vi "GuiUpdate.vi"(7 "GuiRef":T2={"StringOut"=refnum, "AbortOnFail"=refnum, "SN"=refnum, "SN_Length"=refnum, "TestResult"=refnum, "CycleTime"=refnum, "ErrorCode"=refnum, "UUTStatus"=refnum, "DataBaseEnable?"=refnum, "DUTModel"=refnum, "FixtureID"=refnum, "OperatorID"=refnum, "SNReady"=refnum, "StopSlot"=refnum, "NextStep"=refnum, "PassYeild"=refnum, "Failed"=refnum, "Passed"=refnum, "Tested"=refnum, "TestItemsCtl"={"StepName"="", "TestEnable"=FALSE, "LoopCount"=0, "StopOnFail"=FALSE, "Index"=0, "TestName"="", "通道"="", "参数"="", "TimeStart"=0}, "ProcessBar"=refnum, "Slot"=enum."Slot1", "Row"=3, "States"=refnum, "TestMode"=refnum, "循环次数-DUT"=refnum, "波形图"=refnum, "产品型号"=refnum, "子面板"=refnum, "测试失败项目"=refnum, "测试结果"=refnum, "DUT"=refnum, "Starttime"=refnum, "SlotReady"=refnum, "版本信息"=refnum, "WIFI_1"=refnum, "WIFI_2"=refnum, "直通率"=refnum, "卡1开卡结果"=refnum, "卡2开卡结果"=refnum}, 8 "error in":errorcluster, 9 "States":T1=enum."PostUUT") -> (0 "error out":errorcluster, 2 "PASS/FAIL":bool)   [LabVIEW 2013]
uses:
  SysControl/Reference.ctl
  SysControl/TestItemsCTL.ctl
  SysControl/Slot.ctl
  SysControl/States.ctl
  SysControl/LEDState.ctl
  SysControl/Setup.ctl
  SourceCode/GlobalValue.vi
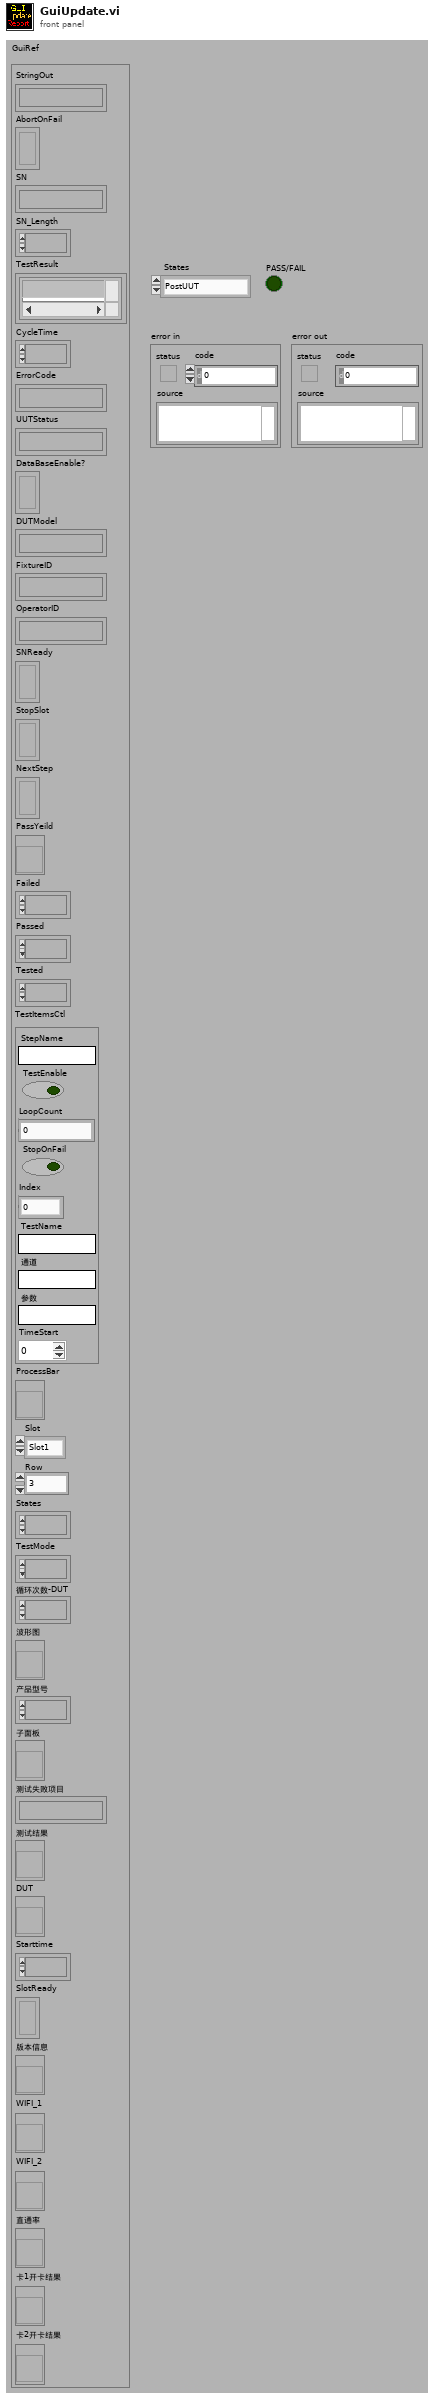
[diagram p1: front panel]
types:
  T1 = typedef "States.ctl" = enum16{"Init", "PreUUT", "Idle", "SetUp", "TestSequence", "PostUUT", "StopTest", "Debug Mode", "Selection Mode", "Loop Mode", "Error", "Wait"}
  T2 = typedef "Reference.ctl" = cluster{"StringOut":refnum<vi>, "AbortOnFail":refnum<vi>, "SN":refnum<vi>, "SN_Length":refnum<vi>, "TestResult":refnum<vi>, "CycleTime":refnum<vi>, "ErrorCode":refnum<vi>, "UUTStatus":refnum<vi>, "DataBaseEnable?":refnum<vi>, "DUTModel":refnum<vi>, "FixtureID":refnum<vi>, "OperatorID":refnum<vi>, "SNReady":refnum<vi>, "StopSlot":refnum<vi>, "NextStep":refnum<vi>, "PassYeild":refnum<vi>, "Failed":refnum<vi>, "Passed":refnum<vi>, "Tested":refnum<vi>, "TestItemsCtl":T3, "ProcessBar":refnum<vi>, "Slot":T4, "Row":u32, "States":refnum<vi>, "TestMode":refnum<vi>, "循环次数-DUT":refnum<vi>, "波形图":refnum<vi>, "产品型号":refnum<vi>, "子面板":refnum<vi>, "测试失败项目":refnum<vi>, "测试结果":refnum<vi>, "DUT":refnum<vi>, "Starttime":refnum<vi>, "SlotReady":refnum<vi>, "版本信息":refnum<vi>, "WIFI_1":refnum<vi>, "WIFI_2":refnum<vi>, "直通率":refnum<vi>, "卡1开卡结果":refnum<vi>, "卡2开卡结果":refnum<vi>}
  T3 = typedef "TestItemsCTL.ctl" = cluster{"StepName":string, "TestEnable":bool, "LoopCount":i32, "StopOnFail":bool, "Index":u32, "TestName":string, "通道":string, "参数":string, "TimeStart":u32}
  T4 = typedef "Slot.ctl" = enum16{"Slot1", "Slot2", "Slot3", "Slot4"}
  T5 = enum8{"Enabled", "Disabled", "Disabled and Grayed Out"}
  T6 = typedef "LEDState.ctl" = enum16{"默认", "闪烁", "停止闪烁", "真", "假"}
  T7 = typedef "Setup.ctl" = cluster{"TestedNum":u32, "PassedNum":u32, "FailedNum":u32, "Slot1TestedNum":u32, "Slot2TestedNum":u32, "Slot3TestedNum":u32, "Slot4TestedNum":u32, "GuiVer":string, "LimitFileVer":string, "Login Name":string, "Password":string, "SN_Head":string, "SN_Length":i32, "AbortOnFail":bool, "DataBaseEnable?":bool, "FixtureID":string, "ShowSkipStep?":bool}
  T8 = typedef "TestMode.ctl" = enum16{"Production Mode", "Selection Mode", "Debug Mode", "Loop Mode", "Stop Test"}
  T9 = enum16{"Production Mode", "Selection Mode", "Debug Mode", "Loop Mode", "Stop Test"}
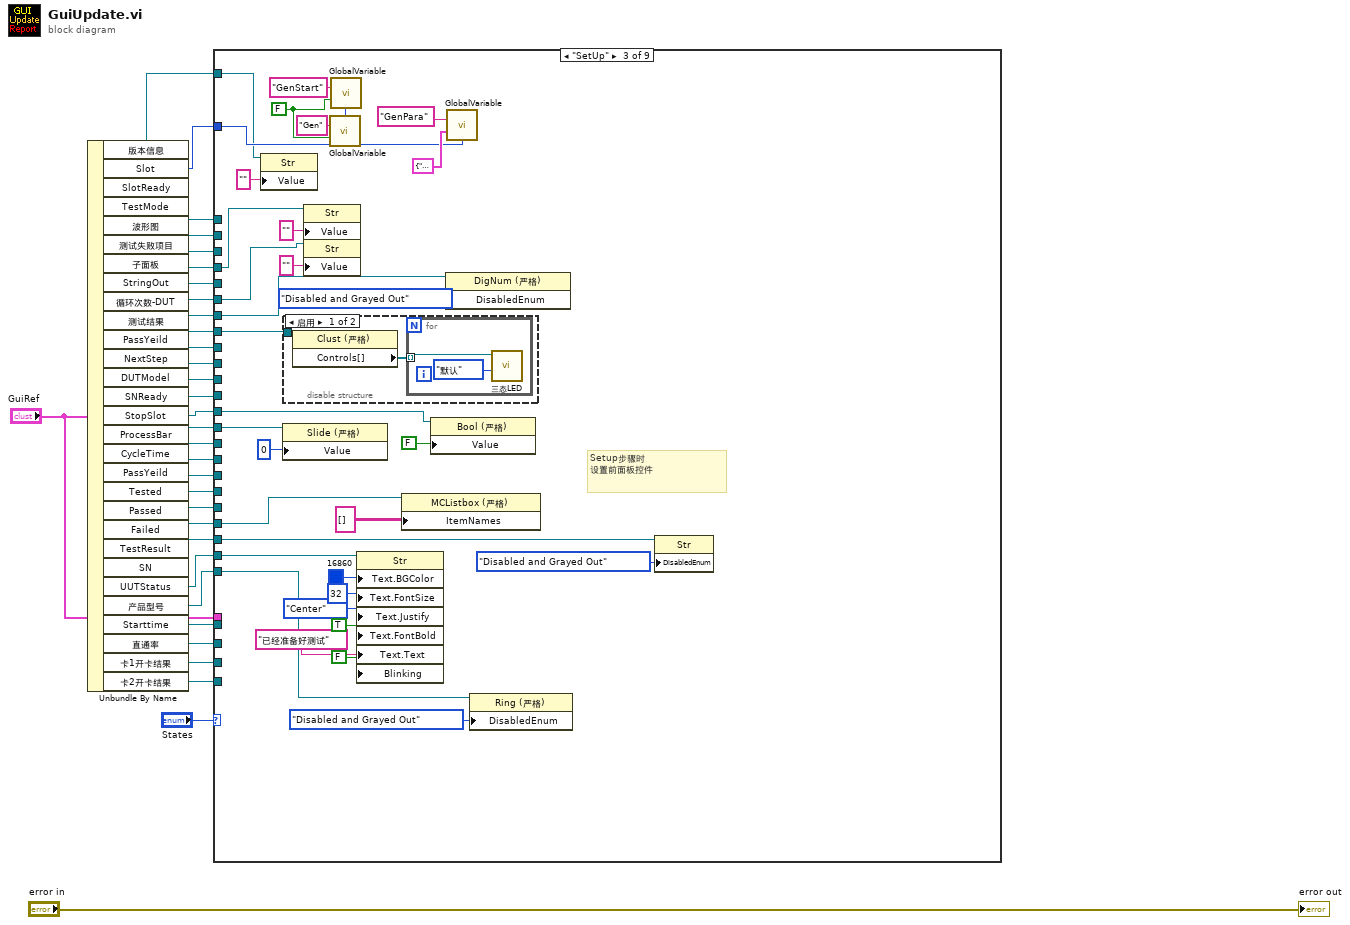
[diagram p0: block diagram]
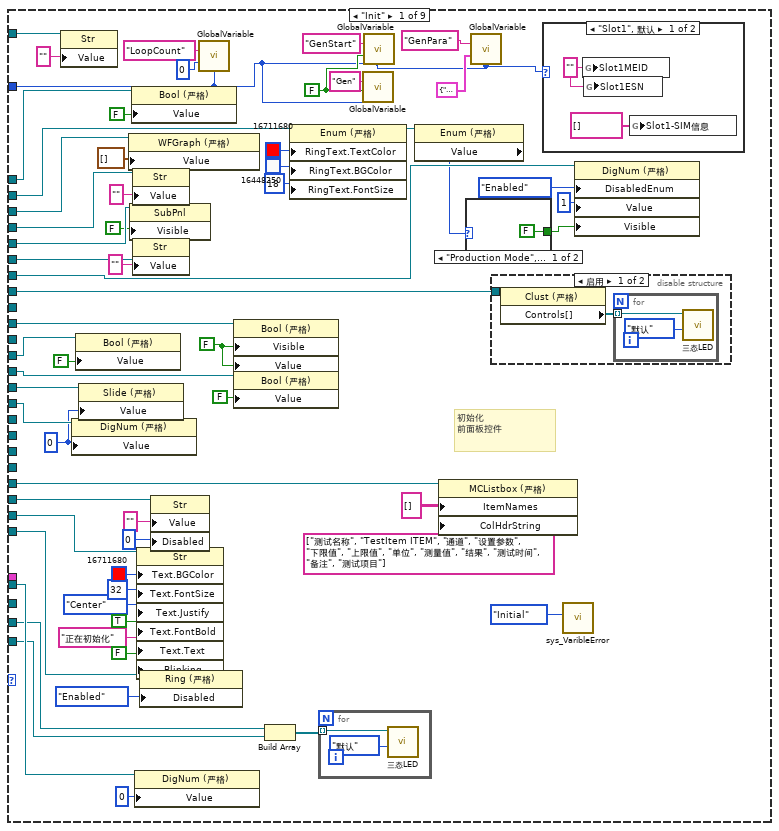
[diagram p2: hidden frame]
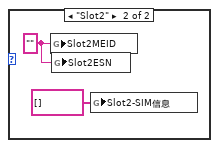
[diagram p3: hidden frame]
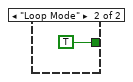
[diagram p4: hidden frame]
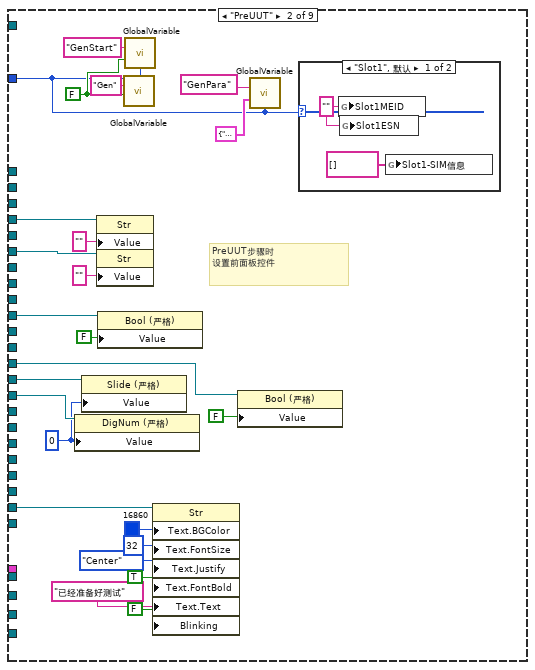
[diagram p6: hidden frame]
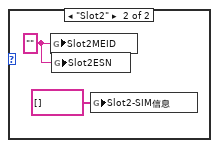
[diagram p7: hidden frame]
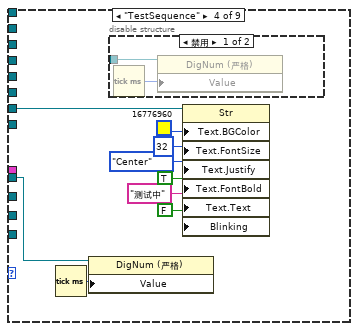
[diagram p9: hidden frame]
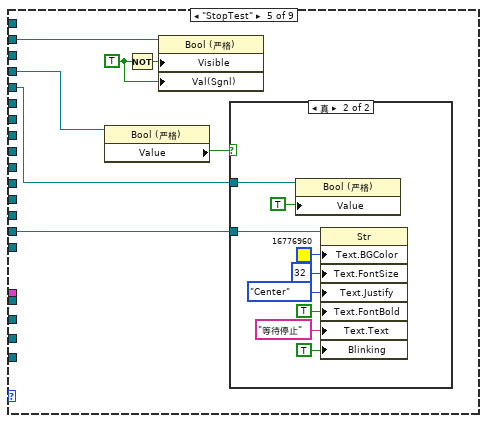
[diagram p11: hidden frame]
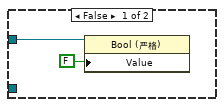
[diagram p12: hidden frame]
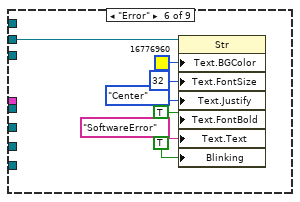
[diagram p13: hidden frame]
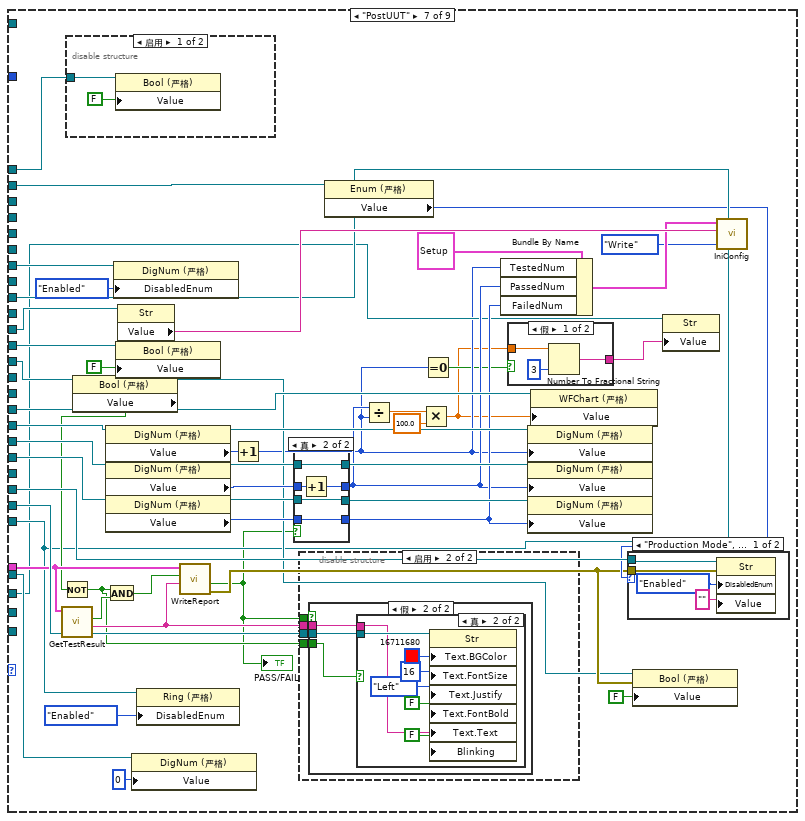
[diagram p14: hidden frame]
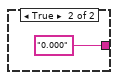
[diagram p15: hidden frame]
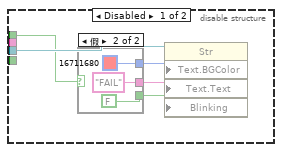
[diagram p18: hidden frame]
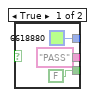
[diagram p19: hidden frame]
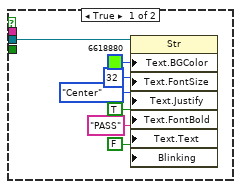
[diagram p20: hidden frame]
diagram:
  n1 = Unbundle By Name("GuiRef") -> ("版本信息"=w4:refnum<vi>, "Slot"=w5:T4, "SlotReady"=w6:refnum<vi>, "TestMode"=w8:refnum<vi>, "波形图"=w9:refnum<vi>, "测试失败项目"=w10:refnum<vi>, "子面板"=w11:refnum<vi>, "StringOut"=w12:refnum<vi>, "循环次数-DUT"=w15:refnum<vi>, "测试结果"=w16:refnum<vi>, "PassYeild"=w18:refnum<vi>, "NextStep"=w19:refnum<vi>, "DUTModel"=w21:refnum<vi>, "SNReady"=w24:refnum<vi>, "StopSlot"=w14:refnum<vi>, "ProcessBar"=w23:refnum<vi>, "CycleTime"=w22:refnum<vi>, "PassYeild"=w28:refnum<vi>, "Tested"=w27:refnum<vi>, "Passed"=w26:refnum<vi>, "Failed"=w25:refnum<vi>, "TestResult"=w30:refnum<vi>, "SN"=w32:refnum<vi>, "UUTStatus"=w31:refnum<vi>, "产品型号"=w13:refnum<vi>, "Starttime"=w7:refnum<vi>, "直通率"=w3:refnum<vi>, "卡1开卡结果"=w2:refnum<vi>, "卡2开卡结果"=w1:refnum<vi>)
  n2 = case shown="\"SetUp\"" "States" {
    tunnel: w32 -> [w91 _ w160 _ _ _ w231 _ _]
    tunnel: w31 -> [w64 w117 w146 w172 w187 w199 w256 _ w340]
    tunnel: w30 -> [w84 _ w163 _ _ _ _ _ _]
    tunnel: w28 -> [_ _ _ _ _ _ w242 _ w321]
    tunnel: w27 -> [_ _ _ _ _ _ w254 _ w337]
    tunnel: w26 -> [_ _ _ _ _ _ w253 _ w336]
    tunnel: w25 -> [_ _ _ _ _ _ w255 _ w338]
    tunnel: w23 -> [w90 w128 w165 _ _ _ _ _ _]
    tunnel: w22 -> [w89 w127 _ _ _ _ _ _ _]
    tunnel: w24 -> [w87 _ _ _ w182 _ w241 _ w319]
    tunnel: w21 -> [_ _ _ _ _ _ w240 _ _]
    tunnel: "GuiRef" -> [_ _ _ _ _ _ w233 _ w318]
    tunnel: w19 -> [w86 w114 _ _ w185 _ _ _ _]
    tunnel: w18 -> [_ _ _ _ _ _ w232 _ _]
    tunnel: w16 -> [w73 _ w158 _ _ _ _ _ _]
    tunnel: w15 -> [w81 _ w162 _ _ _ w230 _ _]
    tunnel: w14 -> [w80 w112 w142 _ w183 _ w228 _ _]
    tunnel: w13 -> [w78 _ w157 _ _ _ w212 _ _]
    tunnel: w12 -> [w76 w124 w155 _ _ _ _ _ _]
    tunnel: w11 -> [w75 _ _ _ _ _ _ _ _]
    tunnel: w10 -> [w71 w122 w153 _ _ _ _ _ _]
    tunnel: w9 -> [w62 _ _ _ _ _ _ _ _]
    tunnel: w8 -> [w57 _ _ _ _ _ w221 _ _]
    tunnel: w7 -> [w54 _ _ w170 _ _ w226 _ _]
    tunnel: w6 -> [w49 _ _ _ _ _ w222 _ w316]
    tunnel: w5 -> [w38 w106 w136 _ _ _ _ _ _]
    tunnel: w4 -> [w37 _ w134 _ _ _ _ _ _]
    tunnel: w3 -> [_ _ _ _ _ _ w210 _ _]
    tunnel: w2 -> [w34 _ _ _ _ _ _ _ _]
    tunnel: w1 -> [w33 _ _ _ _ _ _ _ _]
    frame "Init" {
      w44 = FALSE ("Value")
      w56 = FALSE ("可见")
      w88 = 0 ("Value")
      # "初始化\n前面板控件"
      n3 = property class="Str"(reference=w37, "Value"="" ("值")) -> ()  [unwired: 1 in, 2 out]
      n4 = property class="DigNum (严格)"(reference=w89, "Value"=w88) -> ()  [unwired: 1 in, 2 out]
      n5 = property class="Bool (严格)"(reference=w87, "Value"=FALSE) -> ()  [unwired: 1 in, 2 out]
      n6 = property class="Slide (严格)"(reference=w90, "Value"=w88) -> ()  [unwired: 1 in, 2 out]
      n7 = property class="WFGraph (严格)"(reference=w62, "Value"=waveform(dbl)[] [] ("Fail项波形图2")) -> ()  [unwired: 1 in, 2 out]
      n8 = property class="SubPnl"(reference=w75, "Visible"=FALSE ("可见")) -> ()  [unwired: 1 in, 2 out]
      n9 = property class="Bool (严格)"(reference=w49, "Value"=FALSE) -> ()  [unwired: 1 in, 2 out]
      n10 = property class="Str"(reference=w71, "Value"="" ("值")) -> ()  [unwired: 1 in, 2 out]
      n11 = property class="Str"(reference=w76, "Value"="" ("值")) -> ()  [unwired: 1 in, 2 out]
      n12 = property class="DigNum (严格)"(reference=w54, "Value"=u32 0 ("值")) -> ()  [unwired: 1 in, 2 out]
      n13 = property on="Property Node" class="Str"(reference=w64, "Text.BGColor"=u32 16711680 ("Color Box 2"), "Text.FontSize"=u32 32 ("文本.字体:字号"), "Text.Justify"=enum16{"Left", "Center", "Right"}."Center" ("文本.调整"), "Text.FontBold"=TRUE ("文本.字体:粗体"), "Text.Text"="正在初始化", "Blinking"=FALSE) -> ()  [unwired: 1 in, 2 out]
      n14 = property class="Ring (严格)"(reference=w78, "Disabled"=T5."Enabled" ("禁用")) -> ()  [unwired: 1 in, 2 out]
      n15 = property class="Str"(reference=w91, "Value"="", "Disabled"=u8 0) -> ()  [unwired: 1 in, 2 out]
      n16 = call "GlobalVariable.vi"("Name"="LoopCount", "ValueIn"=0 ("值"), "Slot"=w38) -> ()  [unwired: 9 in, 4 out]
      n17 = property class="Bool (严格)"(reference=w86, "Visible"=w56, "Value"=w56) -> ()  [unwired: 1 in, 2 out]
      n18 = property class="Bool (严格)"(reference=w80, "Value"=FALSE) -> ()  [unwired: 1 in, 2 out]
      n19 = Build Array(w34, w33) -> (w35:refnum<vi>[])
      n20 = property on="属性节点" class="Enum (严格)"(reference=w57, "RingText.TextColor"=u32 16711680 ("Color Box"), "RingText.BGColor"=u32 16448250 ("Color Box"), "RingText.FontSize"=u32 18 ("下拉列表文本.字体:字号")) -> (reference out=w43:refnum<vi>)  [unwired: 1 in, 1 out]
      n21 = for "For循环" {
        tunnel: w35 -> [w94] mode=indexing
        n22 = call "三态LED.vi"("State"=LEDState."默认", "Ctl引用句柄"=w94) -> ()  [unwired: 4 in, 2 out]
      }
      n23 = call "GlobalVariable.vi"("Name"="Gen", "ValueIn"=w44, "Slot"=w38) -> ()  [unwired: 9 in, 4 out]
      n24 = call "GlobalVariable.vi"("Name"="GenStart", "ValueIn"=w44, "Slot"=w38) -> ()  [unwired: 9 in, 4 out]
      n25 = property on="属性节点" class="Enum (严格)"(reference=w43) -> ("Value"=w42:T8)  [unwired: 1 in, 2 out]
      n26 = property class="MCListbox (严格)"(reference=w84, "ItemNames"=string[][] [] ("项名"), "ColHdrString"=string[] ["测试名称", "TestItem ITEM", "通道", "设置参数", "下限值", "上限值", "单位", "测量值", "结果", "测试时间", "备注", "测试项目"] ("列首字符串[]")) -> ()  [unwired: 1 in, 2 out]
      n27 = case shown="\"Production Mode\", 默认" w42 {
        tunnel: [FALSE ("可见") TRUE ("可见")] -> w41
        frame "Production Mode", Default {
        }
        frame "Loop Mode" {
        }
      }
      n28 = call "GlobalVariable.vi"("Name"="GenPara", "ValueIn"=cluster{"CH":tag, "Freq":dbl, "AMP":dbl} {"CH"="Dev1/ao1", "Freq"=0.0, "AMP"=0.0} ("Paras 2"), "Slot"=w38) -> ()  [unwired: 9 in, 4 out]
      n29 = disable-structure shown="启用" {
        disable-tunnel: w73 -> [w103 _]
        frame Enabled {
          n30 = property class="Clust (严格)"(reference=w103) -> ("Controls[]"=w102:refnum<vi>[])  [unwired: 1 in, 2 out]
          n31 = for "For循环" {
            tunnel: w102 -> [w104] mode=indexing
            n32 = call "三态LED.vi"("State"=LEDState."默认", "Ctl引用句柄"=w104) -> ()  [unwired: 4 in, 2 out]
          }
        }
        frame Disabled {
        }
      }
      n33 = case shown="\"Slot1\", 默认" w38 {
        frame "Slot1", Default {
          w97 = "" ("Slot2MEID")
          n34 = global write "GlobalValue.vi" "Slot1MEID"(w97) -> ()
          n35 = global write "GlobalValue.vi" "Slot1ESN"(w97) -> ()
          n36 = global write "GlobalValue.vi" "Slot1-SIM信息"(string[] [] ("Slot2-SIM信息")) -> ()
        }
        frame "Slot2" {
          w99 = "" ("Slot2MEID")
          n37 = global write "GlobalValue.vi" "Slot2MEID"(w99) -> ()
          n38 = global write "GlobalValue.vi" "Slot2ESN"(w99) -> ()
          n39 = global write "GlobalValue.vi" "Slot2-SIM信息"(string[] [] ("Slot2-SIM信息")) -> ()
        }
      }
      n40 = call "sys_VaribleError.vi"("Operation"=enum16{"Initial", "Collect"}."Initial") -> ()  [unwired: 10 in, 1 out]
      n41 = property class="DigNum (严格)"(reference=w81, "DisabledEnum"=T5."Enabled" ("禁用"), "Value"=1 ("值"), "Visible"=w41) -> ()  [unwired: 1 in, 2 out]
    }
    frame "PreUUT" {
      w109 = FALSE ("Value")
      w126 = 0 ("Value")
      # "PreUUT步骤时\n设置前面板控件"
      n42 = property class="DigNum (严格)"(reference=w127, "Value"=w126) -> ()  [unwired: 1 in, 2 out]
      n43 = property class="Slide (严格)"(reference=w128, "Value"=w126) -> ()  [unwired: 1 in, 2 out]
      n44 = property class="Str"(reference=w122, "Value"="" ("值")) -> ()  [unwired: 1 in, 2 out]
      n45 = property class="Str"(reference=w124, "Value"="" ("值")) -> ()  [unwired: 1 in, 2 out]
      n46 = property class="Bool (严格)"(reference=w114, "Value"=FALSE) -> ()  [unwired: 1 in, 2 out]
      n47 = call "GlobalVariable.vi"("Name"="Gen", "ValueIn"=w109) -> ()  [unwired: 10 in, 4 out]
      n48 = call "GlobalVariable.vi"("Name"="GenStart", "ValueIn"=w109, "Slot"=w106) -> ()  [unwired: 9 in, 4 out]
      n49 = property on="Property Node" class="Str"(reference=w117, "Text.BGColor"=u32 16860 ("Color Box 2"), "Text.FontSize"=u32 32 ("文本.字体:字号"), "Text.Justify"=enum16{"Left", "Center", "Right"}."Center" ("文本.调整"), "Text.FontBold"=TRUE ("文本.字体:粗体"), "Text.Text"="已经准备好测试", "Blinking"=FALSE) -> ()  [unwired: 1 in, 2 out]
      n50 = property class="Bool (严格)"(reference=w112, "Value"=FALSE) -> ()  [unwired: 1 in, 2 out]
      n51 = call "GlobalVariable.vi"("Name"="GenPara", "ValueIn"=cluster{"CH":tag, "Freq":dbl, "AMP":dbl} {"CH"="Dev1/ao1", "Freq"=0.0, "AMP"=0.0} ("Paras 2"), "Slot"=w106) -> ()  [unwired: 9 in, 4 out]
      n52 = case shown="\"Slot1\", 默认" w106 {
        frame "Slot1", Default {
          w131 = "" ("Slot2MEID")
          n53 = global write "GlobalValue.vi" "Slot1MEID"(w131) -> ()
          n54 = global write "GlobalValue.vi" "Slot1ESN"(w131) -> ()
          n55 = global write "GlobalValue.vi" "Slot1-SIM信息"(string[] [] ("Slot2-SIM信息")) -> ()
        }
        frame "Slot2" {
          w133 = "" ("Slot2MEID")
          n56 = global write "GlobalValue.vi" "Slot2MEID"(w133) -> ()
          n57 = global write "GlobalValue.vi" "Slot2ESN"(w133) -> ()
          n58 = global write "GlobalValue.vi" "Slot2-SIM信息"(string[] [] ("Slot2-SIM信息")) -> ()
        }
      }
    }
    frame "SetUp" {
      w139 = FALSE ("Value")
      # "Setup步骤时\n设置前面板控件"
      n59 = property class="Str"(reference=w134, "Value"="" ("值")) -> ()  [unwired: 1 in, 2 out]
      n60 = property class="Slide (严格)"(reference=w165, "Value"=0) -> ()  [unwired: 1 in, 2 out]
      n61 = disable-structure shown="启用" {
        disable-tunnel: w158 -> [w167 _]
        frame Enabled {
          n62 = property class="Clust (严格)"(reference=w167) -> ("Controls[]"=w166:refnum<vi>[])  [unwired: 1 in, 2 out]
          n63 = for "For循环" {
            tunnel: w166 -> [w168] mode=indexing
            n64 = call "三态LED.vi"("State"=LEDState."默认", "Ctl引用句柄"=w168) -> ()  [unwired: 4 in, 2 out]
          }
        }
        frame Disabled {
        }
      }
      n65 = property class="Str"(reference=w153, "Value"="" ("值")) -> ()  [unwired: 1 in, 2 out]
      n66 = property class="Str"(reference=w155, "Value"="" ("值")) -> ()  [unwired: 1 in, 2 out]
      n67 = call "GlobalVariable.vi"("Name"="Gen", "ValueIn"=w139, "Slot"=w136) -> ()  [unwired: 9 in, 4 out]
      n68 = call "GlobalVariable.vi"("Name"="GenStart", "ValueIn"=w139, "Slot"=w136) -> ()  [unwired: 9 in, 4 out]
      n69 = property on="Property Node" class="Str"(reference=w146, "Text.BGColor"=u32 16860 ("Color Box 2"), "Text.FontSize"=u32 32 ("文本.字体:字号"), "Text.Justify"=enum16{"Left", "Center", "Right"}."Center" ("文本.调整"), "Text.FontBold"=TRUE ("文本.字体:粗体"), "Text.Text"="已经准备好测试", "Blinking"=FALSE) -> ()  [unwired: 1 in, 2 out]
      n70 = property class="MCListbox (严格)"(reference=w163, "ItemNames"=string[][] [] ("项名")) -> ()  [unwired: 1 in, 2 out]
      n71 = property class="Bool (严格)"(reference=w142, "Value"=FALSE) -> ()  [unwired: 1 in, 2 out]
      n72 = property class="DigNum (严格)"(reference=w162, "DisabledEnum"=T5."Disabled and Grayed Out" ("禁用")) -> ()  [unwired: 1 in, 2 out]
      n73 = call "GlobalVariable.vi"("Name"="GenPara", "ValueIn"=cluster{"CH":tag, "Freq":dbl, "AMP":dbl} {"CH"="Dev1/ao1", "Freq"=0.0, "AMP"=0.0} ("Paras 2"), "Slot"=w136) -> ()  [unwired: 9 in, 4 out]
      n74 = property class="Ring (严格)"(reference=w157, "DisabledEnum"=T5."Disabled and Grayed Out" ("禁用")) -> ()  [unwired: 1 in, 2 out]
      n75 = property class="Str"(reference=w160, "DisabledEnum"=T5."Disabled and Grayed Out" ("禁用")) -> ()  [unwired: 1 in, 2 out]
    }
    frame "TestSequence" {
      n76 = Tick Count (ms)() -> (millisecond timer value=w171:u32)
      n77 = property class="DigNum (严格)"(reference=w170, "Value"=w171) -> ()  [unwired: 1 in, 2 out]
      n78 = disable-structure shown="禁用" {
        disable-tunnel: _ -> [w180 _]
        frame Disabled {
          n79 = Tick Count (ms)() -> (millisecond timer value=w179:u32)
          n80 = property on="Property Node" class="DigNum (严格)"(reference=w180, "Value"=w179) -> ()  [unwired: 1 in, 2 out]
        }
        frame Enabled {
        }
      }
      n81 = property on="Property Node" class="Str"(reference=w172, "Text.BGColor"=u32 16776960 ("Color Box 2"), "Text.FontSize"=u32 32 ("文本.字体:字号"), "Text.Justify"=enum16{"Left", "Center", "Right"}."Center" ("文本.调整"), "Text.FontBold"=TRUE ("文本.字体:粗体"), "Text.Text"="测试中", "Blinking"=FALSE) -> ()  [unwired: 1 in, 2 out]
    }
    frame "StopTest" {
      w184 = TRUE
      n82 = property class="Bool (严格)"(reference=w182) -> ("Value"=w181:bool)  [unwired: 1 in, 2 out]
      n83 = Not(x=w184) -> (.not. x?=w186:bool)
      n84 = property on="属性节点" class="Bool (严格)"(reference=w185, "Visible"=w186, "Val(Sgnl)"=w184) -> ()  [unwired: 1 in, 2 out]
      n85 = case shown="真" w181 {
        tunnel: w187 -> [_ w192]
        tunnel: w183 -> [w189 w191]
        frame False {
          n86 = property class="Bool (严格)"(reference=w189, "Value"=FALSE ("值")) -> ()  [unwired: 1 in, 2 out]
        }
        frame True {
          n87 = property class="Bool (严格)"(reference=w191, "Value"=TRUE ("值")) -> ()  [unwired: 1 in, 2 out]
          n88 = property on="Property Node" class="Str"(reference=w192, "Text.BGColor"=u32 16776960 ("Color Box 2"), "Text.FontSize"=u32 32 ("文本.字体:字号"), "Text.Justify"=enum16{"Left", "Center", "Right"}."Center" ("文本.调整"), "Text.FontBold"=TRUE ("文本.字体:粗体"), "Text.Text"="等待停止", "Blinking"=TRUE) -> ()  [unwired: 1 in, 2 out]
        }
      }
    }
    frame "Error" {
      n89 = property on="Property Node" class="Str"(reference=w199, "Text.BGColor"=u32 16776960 ("Color Box 2"), "Text.FontSize"=u32 32 ("文本.字体:字号"), "Text.Justify"=enum16{"Left", "Center", "Right"}."Center" ("文本.调整"), "Text.FontBold"=TRUE ("文本.字体:粗体"), "Text.Text"="SoftwareError", "Blinking"=TRUE) -> ()  [unwired: 1 in, 2 out]
    }
    frame "PostUUT" {
      n90 = call "GetTestResult.vi"("GuiRef"=w233) -> ("FailStep"=w227:string, "PASS/FAIL"=w218:bool)  [unwired: 3 in, 6 out]
      n91 = disable-structure shown="启用" {
        disable-tunnel: w222 -> [w265 _]
        frame Enabled {
          n92 = property class="Bool (严格)"(reference=w265, "Value"=FALSE ("值")) -> ()  [unwired: 1 in, 2 out]
        }
        frame Disabled {
        }
      }
      n93 = property class="Bool (严格)"(reference=w228) -> (reference out=w214:refnum<vi>, "Value"=w219:bool)  [unwired: 1 in, 1 out]
      n94 = Not(x=w219) -> (.not. x?=w216:bool)
      n95 = property on="Property Node" class="DigNum (严格)"(reference=w254) -> (reference out=w251:refnum<vi>, "Value"=w252:u32)  [unwired: 1 in, 1 out]
      n96 = property on="Property Node" class="DigNum (严格)"(reference=w253) -> (reference out=w247:refnum<vi>, "Value"=w250:u32)  [unwired: 1 in, 1 out]
      n97 = property on="Property Node" class="DigNum (严格)"(reference=w255) -> (reference out=w246:refnum<vi>, "Value"=w249:u32)  [unwired: 1 in, 1 out]
      n98 = And(x=w216, y=w218) -> (x .and. y?=w217:bool)
      n99 = property class="DigNum (严格)"(reference=w230, "DisabledEnum"=T5."Enabled" ("禁用")) -> ()  [unwired: 1 in, 2 out]
      n100 = property class="Bool (严格)"(reference=w241, "Value"=FALSE ("值")) -> ()  [unwired: 1 in, 2 out]
      n101 = property class="Str"(reference=w240) -> ("Value"=w239:string)  [unwired: 1 in, 2 out]
      n102 = property class="DigNum (严格)"(reference=w226, "Value"=u32 0 ("值")) -> ()  [unwired: 1 in, 2 out]
      n103 = property class="Ring (严格)"(reference=w212, "DisabledEnum"=T5."Enabled" ("禁用")) -> ()  [unwired: 1 in, 2 out]
      n104 = call "WriteReport.vi"("StepName"=w227, "Pass/Fail"=w217, "GuiRef"=w233) -> ("error out"=w215:errorcluster, "DBresult"=w211:bool)  [unwired: 6 in, 1 out]
      "PASS/FAIL" <- w211
      n105 = Increment(x=w252) -> (x+1=w208:u32)
      n106 = case shown="真" w211 {
        tunnel: w250 -> [w308 w315]
        tunnel: [w308 w314] -> w236
        tunnel: w249 -> [w310 w313]
        tunnel: [w309 w313] -> w237
        tunnel: [w307 w312] -> w248
        tunnel: w247 -> [w307 w312]
        tunnel: w246 -> [w306 w311]
        tunnel: [w306 w311] -> w245
        frame False {
          n107 = Increment(x=w310) -> (x+1=w309:u32)
        }
        frame True {
          n108 = Increment(x=w315) -> (x+1=w314:u32)
        }
      }
      n109 = disable-structure shown="启用" {
        disable-tunnel: w256 -> [w269 w280]
        disable-tunnel: w211 -> [w267 w281]
        disable-tunnel: w227 -> [_ w279]
        disable-tunnel: w216 -> [_ w278]
        frame Disabled {
          n110 = case shown="假" w267 {
            tunnel: [FALSE ("Blinking") FALSE ("Blinking")] -> w271
            tunnel: ["PASS" ("Text.Text") "FAIL" ("Text.Text")] -> w270
            tunnel: [u32 6618880 ("Color Box 2") u32 16711680 ("Color Box 2")] -> w268
            frame True {
            }
            frame False {
            }
          }
          n111 = property on="Property Node" class="Str"(reference=w269, "Text.BGColor"=w268, "Text.Text"=w270, "Blinking"=w271) -> ()  [unwired: 1 in, 2 out]
        }
        frame Enabled {
          n112 = case shown="假" w281 {
            tunnel: w280 -> [w284 w291]
            tunnel: w279 -> [_ w290]
            tunnel: w278 -> [_ w289]
            frame True {
              n113 = property on="Property Node" class="Str"(reference=w284, "Text.BGColor"=u32 6618880 ("Color Box 2"), "Text.FontSize"=u32 32 ("文本.字体:字号"), "Text.Justify"=enum16{"Left", "Center", "Right"}."Center" ("文本.调整"), "Text.FontBold"=TRUE ("文本.字体:粗体"), "Text.Text"="PASS", "Blinking"=FALSE) -> ()  [unwired: 1 in, 2 out]
            }
            frame False {
              n114 = case shown="真" w289 {
                tunnel: w291 -> [w292 w300]
                tunnel: w290 -> [_ w299]
                frame False {
                  n115 = property on="Property Node" class="Str"(reference=w292, "Text.BGColor"=u32 16711680 ("Color Box 2"), "Text.FontSize"=u32 32 ("文本.字体:字号"), "Text.Justify"=enum16{"Left", "Center", "Right"}."Center" ("文本.调整"), "Text.FontBold"=FALSE ("文本.字体:粗体"), "Text.Text"="中止测试" ("f"), "Blinking"=FALSE) -> ()  [unwired: 1 in, 2 out]
                }
                frame True {
                  n116 = property on="Property Node" class="Str"(reference=w300, "Text.BGColor"=u32 16711680 ("Color Box 2"), "Text.FontSize"=u32 16 ("文本.字体:字号"), "Text.Justify"=enum16{"Left", "Center", "Right"}."Left" ("文本.调整"), "Text.FontBold"=FALSE ("文本.字体:粗体"), "Text.Text"=w299, "Blinking"=FALSE) -> ()  [unwired: 1 in, 2 out]
                }
              }
            }
          }
        }
      }
      n117 = property class="Enum (严格)"(reference=w221) -> ("Value"=w220:T9)  [unwired: 1 in, 2 out]
      n118 = Divide(x=w236, y=w208) -> (x/y=w244:dbl)
      n119 = Multiply(x=w244, y=100.0) -> (x*y=w206:dbl)
      n120 = Equal To 0?(x=w208) -> (x = 0?=w207:bool)
      n121 = Bundle By Name(cluster=T7 {"TestedNum"=10, "PassedNum"=5, "FailedNum"=5, "Slot1TestedNum"=10, "Slot2TestedNum"=10, "Slot3TestedNum"=10, "Slot4TestedNum"=10, "GuiVer"="1.0", "LimitFileVer"="1.0", "Login Name"="", "Password"="", "SN_Head"="0", "SN_Length"=1, "AbortOnFail"=FALSE, "DataBaseEnable?"=FALSE, "FixtureID"="", "ShowSkipStep?"=FALSE} ("IN 2"), "TestedNum"=w208, "PassedNum"=w236, "FailedNum"=w237) -> (w235:T7)
      n122 = case shown="假" w207 {
        tunnel: [w258 "0.000"] -> w209
        tunnel: w206 -> [w257 _]
        frame False {
          n123 = Number To Fractional String(number=w257, precision (6)=3) -> (F-format string=w258:string)  [unwired: 2 in]
        }
        frame True {
        }
      }
      n124 = property on="Property Node" class="DigNum (严格)"(reference=w251, "Value"=w208) -> ()  [unwired: 1 in, 2 out]
      n125 = property on="Property Node" class="DigNum (严格)"(reference=w248, "Value"=w236) -> ()  [unwired: 1 in, 2 out]
      n126 = property on="Property Node" class="DigNum (严格)"(reference=w245, "Value"=w237) -> ()  [unwired: 1 in, 2 out]
      n127 = property on="Property Node" class="WFChart (严格)"(reference=w242, "Value"=w206) -> ()  [unwired: 1 in, 2 out]
      n128 = case shown="\"Production Mode\", 默认" w220 {
        tunnel: w231 -> [w264 _]
        tunnel: w215 -> [w263 _]
        frame "Production Mode", Default {
          n129 = property class="Str"(reference=w264, error in=w263, "DisabledEnum"=T5."Enabled" ("禁用"), "Value"="" ("值")) -> ()  [unwired: 2 out]
        }
        frame "Loop Mode" {
        }
      }
      n130 = property class="Bool (严格)"(reference=w214, error in=w215, "Value"=FALSE ("Blinking")) -> ()  [unwired: 2 out]
      n131 = property class="Str"(reference=w210, "Value"=w209) -> ()  [unwired: 1 in, 2 out]
      n132 = call "IniConfig.vi"("产品型号"=w212, "PassYeild"=w232, "Operate"=enum16{"Write", "Read"}."Write", "ModelName"=w239, "ConfigIn"=w235) -> ()  [unwired: 1 in, 6 out]
    }
    frame "Wait", Default {
    }
    frame "Loop Mode" {
      n133 = property class="Bool (严格)"(reference=w316, "Value"=TRUE) -> ()  [unwired: 1 in, 2 out]
      n134 = property class="Bool (严格)"(reference=w319, "Value"=TRUE) -> ()  [unwired: 1 in, 2 out]
      n135 = property on="Property Node" class="DigNum (严格)"(reference=w337) -> (reference out=w334:refnum<vi>, "Value"=w335:u32)  [unwired: 1 in, 1 out]
      n136 = property on="Property Node" class="DigNum (严格)"(reference=w336) -> (reference out=w328:refnum<vi>, "Value"=w332:u32)  [unwired: 1 in, 1 out]
      n137 = property on="Property Node" class="DigNum (严格)"(reference=w338) -> (reference out=w327:refnum<vi>, "Value"=w331:u32)  [unwired: 1 in, 1 out]
      n138 = Increment(x=w335) -> (x+1=w325:u32)
      n139 = call "GetTestResult.vi"("GuiRef"=w318) -> ("PASS/FAIL"=w333:bool)  [unwired: 2 in, 8 out]
      n140 = case shown="假" w333 {
        tunnel: w332 -> [w346 w353]
        tunnel: [w346 w352] -> w324
        tunnel: w331 -> [w348 w351]
        tunnel: [w347 w351] -> w330
        tunnel: [w345 w350] -> w329
        tunnel: w328 -> [w345 w350]
        tunnel: w327 -> [w344 w349]
        tunnel: [w344 w349] -> w326
        frame False {
          n141 = Increment(x=w348) -> (x+1=w347:u32)
        }
        frame True {
          n142 = Increment(x=w353) -> (x+1=w352:u32)
        }
      }
      n143 = Divide(x=w324, y=w325) -> (x/y=w323:dbl)
      n144 = case shown="真" w333 {
        tunnel: [FALSE ("Blinking") FALSE ("Blinking")] -> w342
        tunnel: ["PASS" ("Text.Text") "FAIL" ("Text.Text")] -> w341
        tunnel: [u32 6618880 ("Color Box 2") u32 16711680 ("Color Box 2")] -> w339
        frame True {
        }
        frame False {
        }
      }
      n145 = Multiply(x=w323, y=1000.0) -> (x*y=w320:dbl)
      n146 = property on="Property Node" class="Str"(reference=w340, "Text.BGColor"=w339, "Text.Text"=w341, "Blinking"=w342) -> ()  [unwired: 1 in, 2 out]
      n147 = property on="Property Node" class="DigNum (严格)"(reference=w334, "Value"=w325) -> ()  [unwired: 1 in, 2 out]
      n148 = property on="Property Node" class="DigNum (严格)"(reference=w329, "Value"=w324) -> ()  [unwired: 1 in, 2 out]
      n149 = property on="Property Node" class="DigNum (严格)"(reference=w326, "Value"=w330) -> ()  [unwired: 1 in, 2 out]
      n150 = property on="Property Node" class="WFChart (严格)"(reference=w321, "Value"=w320) -> ()  [unwired: 1 in, 2 out]
    }
  }
  "error out" <- "error in"
